vi "Compute Sum of Gates Plot Wrapper.vi"(8 "error in (no error)":errorcluster, 11 "VI in":refnum<vi>) -> (0 "error out":errorcluster)   [LabVIEW 2019]
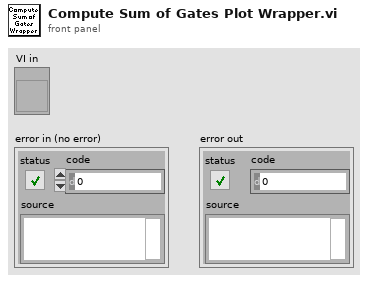
[diagram p1: front panel]
types:
  T1 = typedef "SEPL Parameters.ctl" = cluster{"Display Parameters":T2, "Phasor Parameters":T4, "Decay & IRF Parameters":T7, "Gate Parameters":T9, "Detector Parameters":T11}
  T2 = typedef "Phasor Explorer Display Parameters.ctl" = cluster{"# Points":i32, "Ramp Type":enum16{"Linear", "Logarithmic"}, "Type of Series":T3, "Min tau":dbl[unit], "Max tau":dbl[unit], "Include 0":bool, "Include Infinity":bool}
  T3 = typedef "Type of Series.ctl" = enum16{"1-Exp Decays", "Linear Combination of 1-Exp"}
  T4 = typedef "Phasor Explorer Phasor Parameters.ctl" = cluster{"Harmonic frequency":dbl[unit], "Use f* = 1/D Frequency":bool, "Calibrated Phasor":bool, "Calibration Lifetime":dbl[unit], "Phasor Calculation":T5, "SEPL Type":T6, "# Gates":dbl, "Square Gate Width":dbl[unit], "Show Ticks":bool}
  T5 = typedef "Phasor Calculation Type.ctl" = enum16{"Direct Sum", "Analytical Formula"}
  T6 = typedef "SEPL Type.ctl" = enum16{"UC", "L_N", "L_N[W]"}
  T7 = typedef "Phasor Explorer Decay Parameters.ctl" = cluster{"Lifetime":dbl[unit], "IRF Offset":dbl[unit], "IRF Period":dbl[unit], "Normalized Decays":bool, "IRF Model":T8, "IRF Parameter 1":dbl[unit]}
  T8 = typedef "IRF Model.ctl" = enum16{"Dirac", "Exponential"}
  T9 = typedef "Phasor Explorer Gate Parameters.ctl" = cluster{"First Gate Start":dbl[unit], "Use Gate Center":bool, "Gate Width":dbl[unit], "Gate Step":dbl[unit], "# Gates":dbl, "Gate Type":T10, "Edge Width":dbl[unit], "Top Slope":dbl[unit], "Reversed Sawtooth?":bool, "Analytical Computation":bool, "Integration":enum32{"Item 0", "Item 1"}, "Tolerance":dbl, "# Steps":dbl, "Type of User-defined Function":enum32{"Gate", "IRF"}, "Use Gate Step":bool}
  T10 = typedef "Gate Type.ctl" = enum16{"Square", "Finite Edge Square", "Finite Edge, Tilted Top Square", "Triangle", "Sawtooth", "User-defined"}
  T11 = typedef "Phasor Explorer Detector Parameters.ctl" = cluster{"Frames/Image":i32, "Gates/Frame":i32, "Bits/Frame":i32, "Multiplicity":i32, "Incident Signal":dbl, "Poisson Signal":bool}
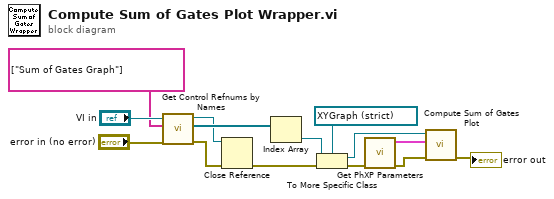
[diagram p0: block diagram]
diagram:
  n1 = call "Get Control Refnums by Names.vi"("error in"="error in (no error)", "Control Labels"=string[] ["Sum of Gates Graph"], "VI  Ref"="VI in") -> ("error out"=w12:errorcluster, "Ctl Refnums"=w14:refnum<vi>[], "VI  Ref (out)"=w7:refnum<vi>)  [unwired: 5 in, 1 out]
  n2 = Close Reference(reference=w7, error in (no error)=w12) -> (error out=w1:errorcluster)
  n3 = Index Array(array=w14) -> (element=w13:refnum<vi>)  [unwired: 1 in]
  n4 = To More Specific Class(target class=refnum<vi> refnum ("Sum of Gates Graph Refnum"), reference=w13, error in=w1) -> (specific class reference=w6:refnum<vi>, error out=w3:errorcluster)
  n5 = call "Get PhXP Parameters.vi"("Error In"=w3) -> ("Error Out"=w2:errorcluster, "Phasor Explorer Parameters"=w4:T1)  [unwired: 7 in, 2 out]
  n6 = call "Compute Sum of Gates Plot.vi"("Error In"=w2, "Phasor Parameters"=w4, "Sum of Gates Graph Refnum"=w6) -> ("Error Out"=→"error out":errorcluster)  [unwired: 7 in, 1 out]
